vi "LaunchGSW__slk_mt.vi"(8 "error in (no error)":errorcluster) -> (0 "error out":errorcluster)   [LabVIEW 2013, in "Lazyboots Menu Tool.lvlib"]
doc: "Lauches GSW agent dynamically."
uses:
  Library/Lazyboots Menu Tool.lvlib
panel:
  # "LaunchGSW__slk_mt.vi\nLauches GSW agent dynamically.\n\nNOTICE -- YOU MUST LEAVE THIS NOTICE IN PLACE.\n\nCopyright (c) 2011, LIANG LIU Shawn.Liu.cn@gmail.com\nAll rights reserved.\n\nRedistribution and use in source and binary forms, with or without modification, are permitted provided that the following conditions are met:\n-Redistributions of source code must retain the above copyright notice, this list of conditions and the following disclaimer.\n-Redistributions in binary form must reproduce the above copyright notice, this list of conditions and the following disclaimer in the documentation and/or other materials provided with the distribution.\n-Neither the name of the eLp nor the names of its contributors may be used to endorse or promote products derived from this software without specific prior written permission.\n\nTHIS SOFTWARE IS PROVIDED BY THE COPYRIGHT HOLDERS AND CONTRIBUTORS \"AS IS\" AND ANY EXPRESS OR IMPLIED WARRANTIES, INCLUDING, BUT NOT LIMITED TO, THE IMPLIED WARRANTIES OF MERCHANTABILITY AND FITNESS FOR A PARTICULAR PURPOSE ARE DISCLAIMED. IN NO EVENT SHALL THE COPYRIGHT HOLDER OR CONTRIBUTORS BE LIABLE FOR ANY DIRECT, INDIRECT, INCIDENTAL, SPECIAL, EXEMPLARY, OR CONSEQUENTIAL DAMAGES (INCLUDING, BUT NOT LIMITED TO, PROCUREMENT OF SUBSTITUTE GOODS OR SERVICES; LOSS OF USE, DATA, OR PROFITS; OR BUSINESS INTERRUPTION) HOWEVER CAUSED AND ON ANY THEORY OF LIABILITY, WHETHER IN CONTRACT, STRICT LIABILITY, OR TORT (INCLUDING NEGLIGENCE OR OTHERWISE) ARISING IN ANY WAY OUT OF THE USE OF THIS SOFTWARE, EVEN IF ADVISED OF THE POSSIBILITY OF SUCH DAMAGE."
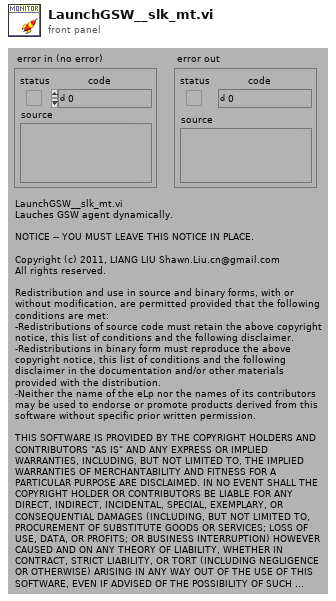
[diagram p1: front panel]
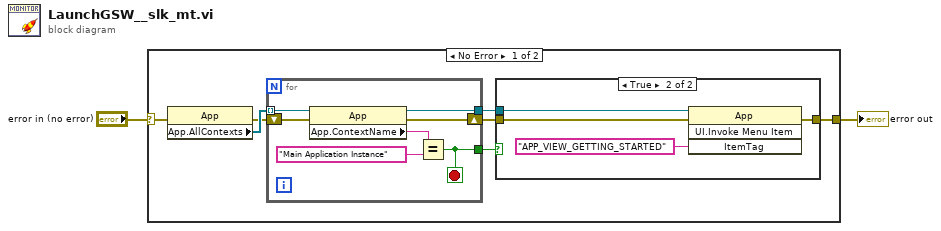
[diagram p0: block diagram]
diagram:
  n1 = case shown="No Error" "error in (no error)" {
    selector: "error in (no error)" -> [w5 w22]
    tunnel: [w4 w22] -> w1
    frame No Error {
      n2 = property class="App"(error in=w5) -> (error out=w3:errorcluster, "App.AllContexts"=w9:refnum<vi>[])  [unwired: 1 in, 1 out]
      n3 = for {
        tunnel: w9 -> [w21] mode=indexing
        shift-right: [w19] -> w7
        shift-left: w3 -> [w20]
        tunnel: [w16] -> w6
        tunnel: [w15] -> w8
        stop <- w15 stop-if-true
        n4 = property class="App"(reference=w21, error in=w20) -> (reference out=w16:refnum<vi>, error out=w19:errorcluster, "App.ContextName"=w18:string)
        n5 = Equal?(x=w18, y="Main Application Instance") -> (x = y?=w15:bool)
      }
      n6 = case shown="True" w8 {
        tunnel: w7 -> [w10 w13]
        tunnel: w6 -> [_ w12]
        tunnel: [w10 w11] -> w4
        frame False {
        }
        frame True {
          n7 = invoke class="App" method="UI.Invoke Menu Item"(reference=w12, error in=w13, "ItemTag"="APP_VIEW_GETTING_STARTED" ("Menu Item Tag")) -> (error out=w11:errorcluster)  [unwired: 1 in, 3 out]
        }
      }
    }
    frame Error {
    }
  }
  "error out" <- w1
